vi "Run all tests CLI.vi"   [LabVIEW 2021]
uses:
  <vilib>/addons/_JKI Toolkits/Caraya/classes/Test Report/Test Report.lvclass
  <vilib>/Wiresmith Technology/G CLI/CLI Class/CLI.lvclass
types:
  T1 = enum32{"Invalid", "Standard", "Closed", "Hidden", "Minimized", "Maximized"}
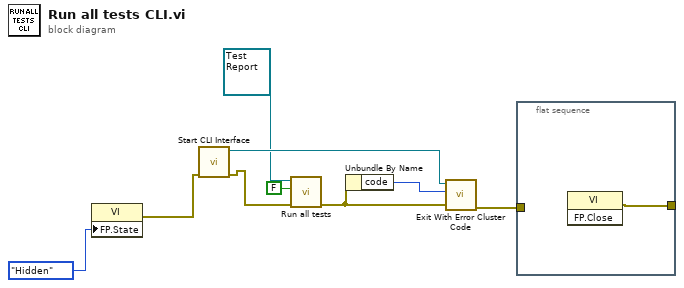
[diagram p0: block diagram]
diagram:
  n1 = property class="VI"("FP.State"=T1."Hidden" ("Front Panel Window:State")) -> (error out=w6:errorcluster)  [unwired: 2 in, 1 out]
  n2 = call <vilib>:"Start CLI Interface.vi"("error in (no error)"=w6) -> ("error out"=w5:errorcluster, "CLI out"=w7:refnum<class "CLI.lvclass">)  [unwired: 7 in, 2 out]
  n3 = call "Run all tests.vi"("error in (no error)"=w5, "Interactive (T)"=FALSE, "Test Report"=refnum<class "Test Report.lvclass"> refnum) -> ("error out"=w2:errorcluster)  [unwired: 7 in, 1 out]
  n4 = Unbundle By Name(w2) -> ("code"=w1:i32)
  n5 = call <vilib>:"Exit With Error Cluster Code.vi"("error in (no error)"=w2, "No Error Code (0)"=w1, "CLI in"=w7) -> ("error out"=w8:errorcluster)  [unwired: 8 in]
  n6 = flat-sequence {
    tunnel: [w10] -> _
    tunnel: w8 -> [_]
    frame #0 {
      n7 = invoke class="VI" method="FP.Close"() -> (error out=w10:errorcluster)  [unwired: 3 in, 2 out]
    }
  }
